vi "GE 5565PIORC.Bit Manipulation.Get Bit (U32).vi"(9 "bit index":i32, 11 "packed value in":u32 format="%016x") -> (2 "bit":bool, 3 "packed value out":u32 format="%016x")   [LabVIEW 2020, in "GE 5565PIORC.lvclass"]
doc: "This VI reads the bit located at <B>bit index</B> in <B>packed value</B>."
uses:
  GE 5565PIORC.lvclass
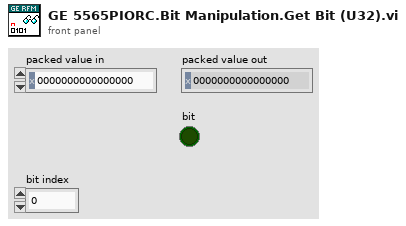
[diagram p1: front panel]
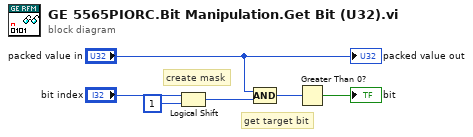
[diagram p0: block diagram]
diagram:
  # "create mask"
  # "get target bit"
  n1 = Logical Shift(y="bit index", x=u32 1) -> (x << y=w5:u32)
  n2 = Compound Arithmetic op=AND("packed value in", w5) -> (w2:u32)
  n3 = Greater Than 0?(x=w2) -> (x > 0?=→"bit":bool)
  "packed value out" <- "packed value in"
